vi "Timer.vi"(11 "State":enum16{"GetTime", "InitTime"}(ring)) -> (3 "Timer (s)":dbl)   [LabVIEW 2020]
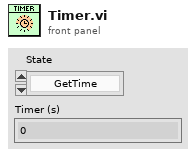
[diagram p1: front panel]
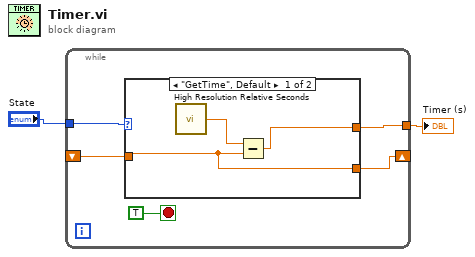
[diagram p0: block diagram]
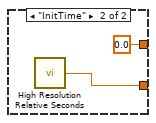
[diagram p2: hidden frame]
diagram:
  n1 = while {
    tunnel: "State" -> [w7]
    shift-right: [w3] -> _
    shift-left: _ -> [w6]
    tunnel: [w4] -> w1
    stop <- TRUE stop-if-true
    n2 = case shown="\"GetTime\", Default" w7 {
      tunnel: [w9 0.0] -> w4
      tunnel: w6 -> [w8 _]
      tunnel: [w8 w11] -> w3
      frame "GetTime", Default {
        n3 = call <vilib>:"High Resolution Relative Seconds.vi"() -> ("relative seconds"=w10:dbl)
        n4 = Subtract(x=w10, y=w8) -> (x-y=w9:dbl)
      }
      frame "InitTime" {
        n5 = call <vilib>:"High Resolution Relative Seconds.vi"() -> ("relative seconds"=w11:dbl)
      }
    }
  }
  "Timer (s)" <- w1
